vi "Validate.vi"(8 "error in (no error)":errorcluster, 11 "MagLabGraph in":refnum<class "XY Plot.lvclass">) -> (0 "error out":errorcluster, 3 "MagLabGraph out":refnum<class "XY Plot.lvclass">)   [LabVIEW 2018, in "XY Plot.lvclass"]
uses:
  XY Plot.lvclass
  XY Plot.lvclass/XY Plot.ctl
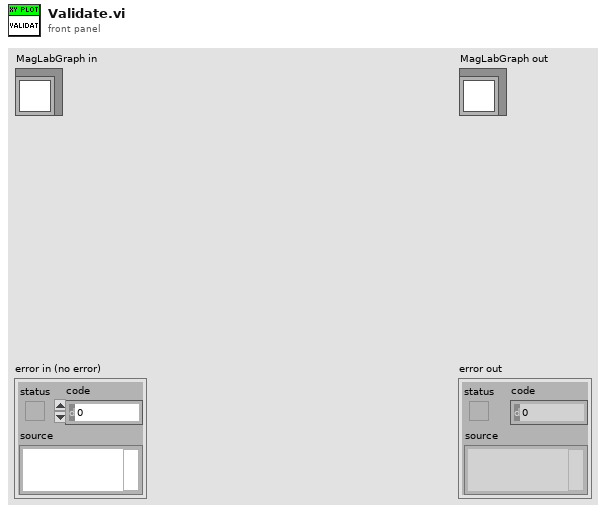
[diagram p1: front panel]
types:
  T1 = cluster{"File Path Control":path, "Group":string, "Channel":string, "Abbreviated":string}[]
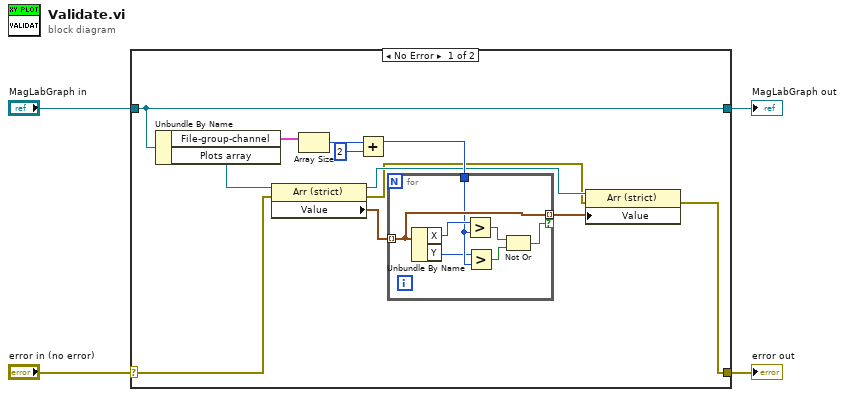
[diagram p0: block diagram]
diagram:
  n1 = case shown="No Error" "error in (no error)" {
    selector: "error in (no error)" -> [w14 w25]
    tunnel: [w5 w25] -> w3
    tunnel: [w16 w24] -> w1
    tunnel: "MagLabGraph in" -> [w16 w24]
    frame No Error {
      n2 = Unbundle By Name(w16) -> ("File-group-channel"=w12:T1, "Plots array"=w15:refnum<vi>)
      n3 = property class="Arr (strict)"(reference=w15, error in=w14) -> (reference out=w7:refnum<vi>, error out=w6:errorcluster, "Value"=w13:cluster{"X":u16, "Y":u16}[])
      n4 = Array Size(array=w12) -> (size(s)=w11:i32)
      n5 = Add(x=w11, y=2) -> (x+y=w10:i32)
      n6 = for {
        tunnel: w13 -> [w21] mode=indexing
        tunnel: w10 -> [w18]
        tunnel: [w21] -> w8 mode=indexing if=w20
        n7 = Unbundle By Name(w21) -> ("X"=w19:u16, "Y"=w17:u16)
        n8 = Greater?(x=w19, y=w18) -> (0:w22:bool)
        n9 = Greater?(x=w17, y=w18) -> (0:w23:bool)
        n10 = Not Or(1:w23, 2:w22) -> (0:w20:bool)
      }
      n11 = property class="Arr (strict)"(reference=w7, error in=w6, "Value"=w8) -> (error out=w5:errorcluster)  [unwired: 1 out]
    }
    frame Error {
    }
  }
  "error out" <- w3
  "MagLabGraph out" <- w1
